vi "Valve Control USB6008.vi"(0 "Port":tag="Dev2/port0", 2 "Mode":enum16{"Read", "Write"}(ring), 5 "Write Val":u8, 11 "error in":errorcluster) -> (6 "Data":u8=255 caption="Data to Write" format="%x", 15 "error out":errorcluster)   [LabVIEW 2016]
doc: "I. Description:\nThis example demonstrates how to write values to a digital output port.\n\nII. Instructions for Running:\n1. Select the digital port on the DAQ device to be written.\n2. Select a value to write.\nNote: The Data to Write control is in hexadecimal.\n\nIII. Block Diagram Steps:\n1. Create a Digital Output channel. Use one channel for all lines. In this case, the port itself acts as an individual channel.\n2. Call the Start VI to start the task.\n3. Write digital port data in a loop until the user hits the stop button or an error occurs. This write VI writes a single sample of digital data on demand, so no timeout is necessary.\n4. Call the Clear Task VI to clear the Task.\n5. Use the popup dialog box to display an error or warning if any.\n\nIV. I/O Connections Overview:\nMake sure your signal output terminals match the Ports I/O Control. In this case wire the item to receive the signal to the first N digital lines on your DAQ Device."
uses:
  <vilib>/DAQmx/read.llb/DAQmx Read (Digital U8 1Chan 1Samp).vi
  <vilib>/DAQmx/write.llb/DAQmx Write (Digital U8 1Chan 1Samp).vi
  <vilib>/DAQmx/create/channels.llb/DAQmx Create Channel (DO-Digital Output).vi
  <vilib>/DAQmx/miscellaneous.llb/DAQmx Fill In Error Info.vi
panel:
  # "For instructions, select Help>>Show Context Help"
  # "Channel Parameters"
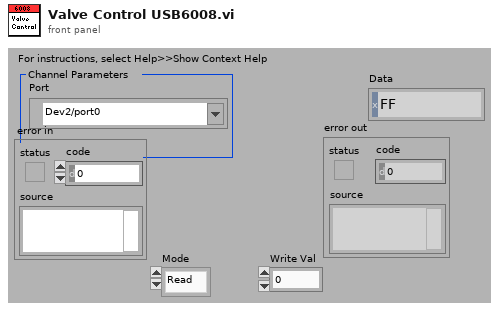
[diagram p1: front panel]
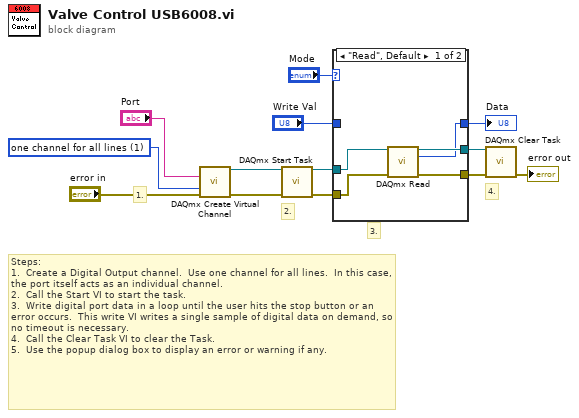
[diagram p0: block diagram]
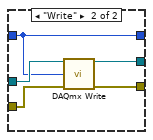
[diagram p2: hidden frame]
diagram:
  w6 = 1 items=["one channel for each line", "one channel for all lines"] ("line grouping")
  # "3."
  # "Steps: \n1.  Create a Digital Output channel.  Use one channel for all lines.  In this case, the port itself acts as an individual channel.\n2.  Call the Start VI to start the task.\n3.  Write digital port data in a loop until the user hits the stop button or an error occurs.  This write VI writes a single sample of digital data on demand, so no timeout is necessary.\n4.  Call the Clear Task VI to clear the Task.\n5.  Use the popup dialog box to display an error or warning if any."
  # "4."
  # "2."
  # "1."
  n1 = call-poly <vilib>:"DAQmx Create Virtual Channel.vi"("lines"="Port", "line grouping"=w6, "error in"="error in") -> ("task out"=w9:refnum<k21>, "error out"=w8:errorcluster)  [unwired: 11 in]
  n2 = call <vilib>:"DAQmx Start Task.vi"("task/channels in"=w9, "error in"=w8) -> ("task out"=w11:refnum<k21>, "error out"=w13:errorcluster)  [unwired: 12 in]
  n3 = case shown="\"Read\", Default" "Mode" {
    tunnel: w13 -> [w16 w23]
    tunnel: [w15 w22] -> w12
    tunnel: w11 -> [w18 w21]
    tunnel: [w17 w20] -> w10
    tunnel: "Write Val" -> [_ w19]
    tunnel: [w14 w19] -> w4
    frame "Read", Default {
      n4 = call-poly <vilib>:"DAQmx Read.vi"("task/channels in"=w18, "error in"=w16) -> ("task out"=w17:refnum<k21>, "data"=w14:u8, "error out"=w15:errorcluster)  [unwired: 11 in]
    }
    frame "Write" {
      n5 = call-poly <vilib>:"DAQmx Write.vi"("task/channels in"=w21, "data"=w19, "error in"=w23) -> ("task out"=w20:refnum<k21>, "error out"=w22:errorcluster)  [unwired: 10 in, 1 out]
    }
  }
  "Data" <- w4
  n6 = call <vilib>:"DAQmx Clear Task.vi"("task in"=w10, "error in"=w12) -> ("error out"=→"error out":errorcluster)  [unwired: 13 in]
